vi "UI.LoadComboBoxes.vi"(8 "error in (no error)":errorcluster, 11 "State Variables":T1) -> (0 "error out":errorcluster)   [LabVIEW 2013, in "Simple Sequence Editor.lvlib"]
uses:
  Simple Sequence Editor.lvlib
  Types/StateVariables.ctl
  Types/ChannelProperties.ctl
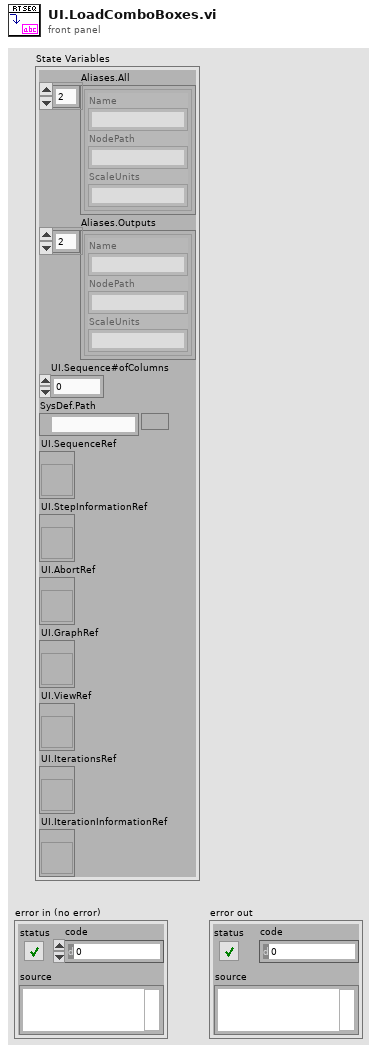
[diagram p1: front panel]
types:
  T1 = typedef "Simple Sequence Editor.lvlib/StateVariables.ctl" = cluster{"Aliases.All":T2[], "Aliases.Outputs":T2[], "UI.Sequence#ofColumns":i32, "SysDef.Path":path, "UI.SequenceRef":refnum<vi>, "UI.StepInformationRef":refnum<vi>, "UI.AbortRef":refnum<vi>, "UI.GraphRef":refnum<vi>, "UI.ViewRef":refnum<vi>, "UI.IterationsRef":refnum<vi>, "UI.IterationInformationRef":refnum<vi>}
  T2 = typedef "Simple Sequence Editor.lvlib/ChannelProperties.ctl" = cluster{"Name":string, "NodePath":string, "ScaleUnits":string}
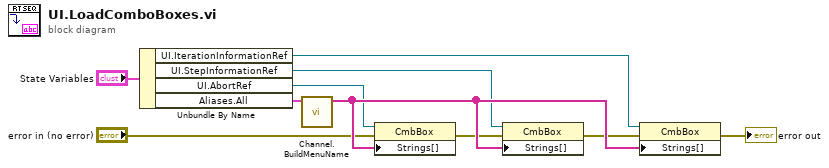
[diagram p0: block diagram]
diagram:
  n1 = Unbundle By Name("State Variables") -> ("UI.IterationInformationRef"=w7:refnum<vi>, "UI.StepInformationRef"=w5:refnum<vi>, "UI.AbortRef"=w3:refnum<vi>, "Aliases.All"=w2:T2[])
  n2 = call "Channel.BuildMenuName.vi"("Aliases"=w2) -> ("Aliases Array"=w10:string[])  [unwired: 10 in]
  n3 = property class="CmbBox"(reference=w3, error in="error in (no error)", "Strings[]"=w10) -> (error out=w4:errorcluster)  [unwired: 1 out]
  n4 = property class="CmbBox"(reference=w5, error in=w4, "Strings[]"=w10) -> (error out=w8:errorcluster)  [unwired: 1 out]
  n5 = property class="CmbBox"(reference=w7, error in=w8, "Strings[]"=w10) -> (error out=→"error out":errorcluster)  [unwired: 1 out]
